vi "Sukh Veer_HWQ2.vi"() -> ()   [LabVIEW 2015]
panel:
  out "Array 2":bool[](array[boolean])=[FALSE, FALSE, TRUE, FALSE, FALSE, TRUE, FALSE, TRUE, TRUE, TRUE, TRUE, FALSE]
  in  "Array":dbl[](array[numeric])=[7.0, 4.0, 11.0, 3.0, 7.0, 65.0, 6.0, 56.0, 67.0, 23.0, 12.0, 9.0]
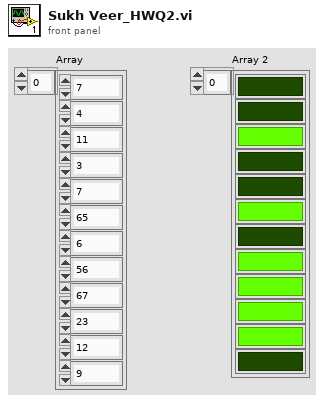
[diagram p1: front panel]
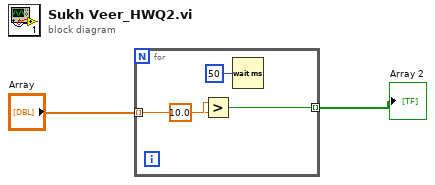
[diagram p0: block diagram]
diagram:
  n1 = for {
    tunnel: "Array" -> [w6] mode=indexing
    tunnel: [w4] -> w1 mode=indexing
    n2 = Greater?(x=w6, y=10.0) -> (0:w4:bool)
    n3 = Wait (ms)(milliseconds to wait=u32 50) -> ()  [unwired: 1 out]
  }
  "Array 2" <- w1
